vi "Write address.vi"(8 "error in (no error)":errorcluster, 10 "address":string="192.168.14.151", 11 "TCPCommClass in":refnum<class "TCPCommClass.lvclass">) -> (0 "error out":errorcluster, 3 "TCPCommClass out":refnum<class "TCPCommClass.lvclass">)   [LabVIEW 2020, in "TCPCommClass.lvclass"]
uses:
  TCPCommClass.lvclass
  TCPCommClass.lvclass/TCPCommClass.ctl
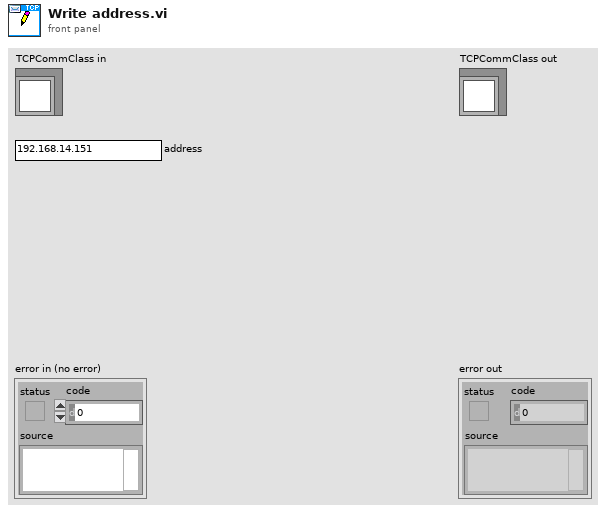
[diagram p1: front panel]
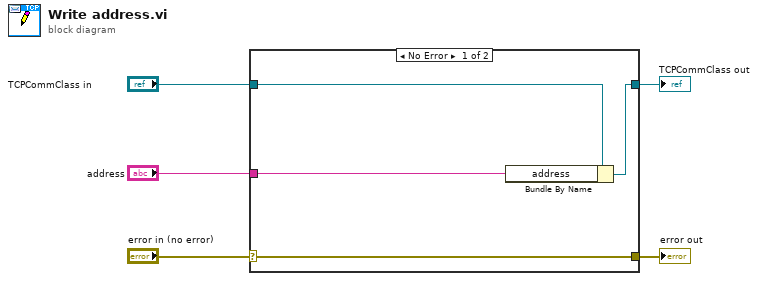
[diagram p0: block diagram]
diagram:
  n1 = case shown="No Error" "error in (no error)" {
    selector: "error in (no error)" -> [w9 w10]
    tunnel: [w9 w10] -> w4
    tunnel: [w7 w11] -> w2
    tunnel: "TCPCommClass in" -> [w8 w11]
    tunnel: "address" -> [w6 _]
    frame No Error {
      n2 = Bundle By Name(cluster=w8, "address"=w6) -> (w7:refnum<class "TCPCommClass.lvclass">)
    }
    frame Error {
    }
  }
  "error out" <- w4
  "TCPCommClass out" <- w2
